vi "Write Outgoing Bytes.vi"(8 "error in (no error)":errorcluster, 9 "timeout ms (2000)":i32=2000, 10 "Bytes":u8[](array[numeric]) format="%08b", 11 "TCPConnection in":refnum<class "TCPConnection.lvclass">) -> (0 "error out":errorcluster, 3 "TCPConnection out":refnum<class "TCPConnection.lvclass">)   [LabVIEW 2013, in "MQTT_TCP.lvlib" / "TCPConnection.lvclass"]
uses:
  TCPConnection.lvclass
  TCPConnection.lvclass/TCPConnection.ctl
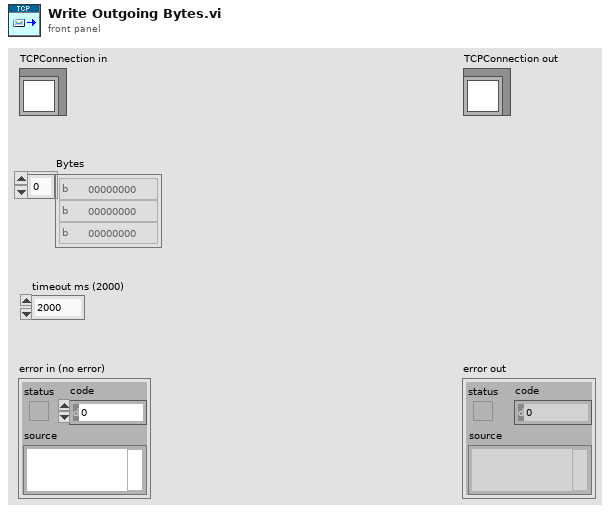
[diagram p1: front panel]
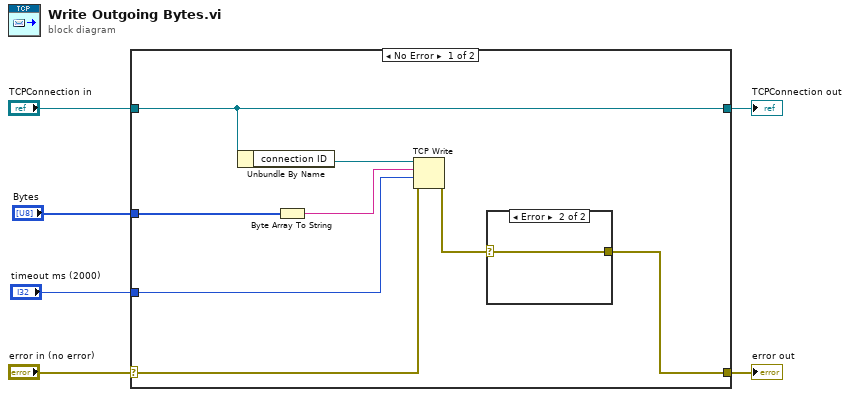
[diagram p0: block diagram]
diagram:
  n1 = case shown="No Error" "error in (no error)" {
    selector: "error in (no error)" -> [w10 w18]
    tunnel: [w8 w18] -> w5
    tunnel: [w14 w17] -> w3
    tunnel: "TCPConnection in" -> [w14 w17]
    tunnel: "Bytes" -> [w12 _]
    tunnel: "timeout ms (2000)" -> [w7 _]
    frame No Error {
      n2 = Unbundle By Name(w14) -> ("connection ID"=w13:refnum<k5>)
      n3 = Byte Array To String(unsigned byte array=w12) -> (string=w11:string)
      n4 = TCP Write(connection ID=w13, data in=w11, error in (no error)=w10, 9:w7) -> (error out=w9:errorcluster)  [unwired: 2 out]
      n5 = case shown="No Error" w9 {
        selector: w9 -> [w15 w16]
        tunnel: [w15 w16] -> w8
        frame No Error {
        }
        frame Error {
        }
      }
    }
    frame Error {
    }
  }
  "error out" <- w5
  "TCPConnection out" <- w3
